vi "Adv_CompareProcesses.vi"(8 "error in (no error)":errorcluster, 9 "AddInProcess Processes New":i32[](array[numeric]), 10 "AddInProcess Processes Old":i32[](array[numeric]), 11 "LightField Automation in":refnum<class "LightField Automation.lvclass">) -> (0 "error out":errorcluster, 2 "New Process":i32, 3 "LightField Automation out":refnum<class "LightField Automation.lvclass">)   [LabVIEW 2015, in "LightField Automation.lvclass"]
uses:
  LightField Automation.lvclass
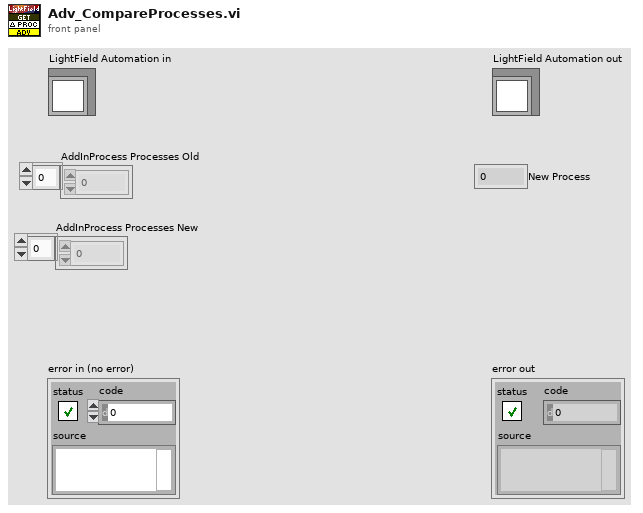
[diagram p1: front panel]
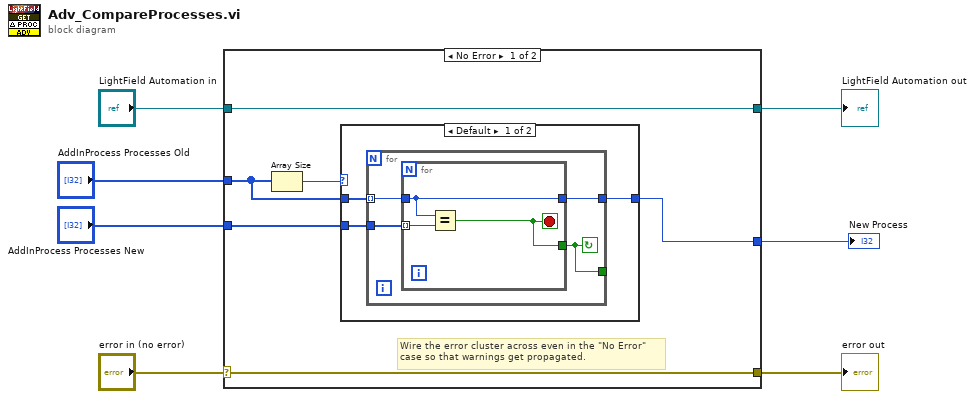
[diagram p0: block diagram]
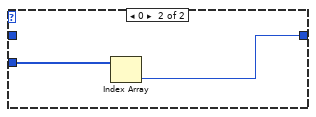
[diagram p2: hidden frame]
diagram:
  n1 = case shown="No Error" "error in (no error)" {
    selector: "error in (no error)" -> [w12 w27]
    tunnel: [w12 w27] -> w6
    tunnel: [w13 w26] -> w4
    tunnel: "LightField Automation in" -> [w13 w26]
    tunnel: "AddInProcess Processes Old" -> [w9 _]
    tunnel: "AddInProcess Processes New" -> [w10 _]
    tunnel: [w8 _] -> w1
    frame No Error {
      # "Wire the error cluster across even in the \"No Error\"\ncase so that warnings get propagated."
      n2 = Array Size(array=w9) -> (size(s)=w11:i32)
      n3 = case shown="Default" w11 {
        tunnel: w10 -> [w15 w25]
        tunnel: w9 -> [w16 _]
        tunnel: [w14 w24] -> w8
        frame Default {
          n4 = for {
            tunnel: w16 -> [w19] mode=indexing
            tunnel: w15 -> [w20]
            tunnel: [w18] -> w14
            tunnel: [w17] -> _
            stop <- w17 continue-if-true
            n5 = for {
              tunnel: w20 -> [w23] mode=indexing
              tunnel: w19 -> [w21]
              tunnel: [w21] -> w18
              tunnel: [w22] -> w17
              stop <- w22 stop-if-true
              n6 = Equal?(x=w21, y=w23) -> (x = y?=w22:bool)
            }
          }
        }
        frame 0 {
          n7 = Index Array(array=w25) -> (element=w24:i32)  [unwired: 1 in]
        }
      }
    }
    frame Error {
    }
  }
  "error out" <- w6
  "LightField Automation out" <- w4
  "New Process" <- w1
